vi "ColorSensor.vi"() -> ()   [LabVIEW 2016, in "ENED1100-UCBA-Sensor-Motor-Testing.lvrbt"]
uses:
  ENED1100-UCBA-Sensor-Motor-Testing.lvrbt
  <vilib>/NXT/Subs/LVHSConnector.ctl
  <vilib>/NXT/LegoClasses/BrickReference/BrickReference.lvclass
  <vilib>/NXT/Block Support/NXT_InputPort.ctl
  <vilib>/NXT/Subs/ColorSensorColors.ctl
  <vilib>/NXT/Dual Mode Library/Sensors/EV3_Color_Color.vi
panel:
  out "NXT/EV3 2":T1
  out "Detected Color":T2
  in  "Select Port Here":T3 items=["Port 1", "Port 2", "Port 3", "Port 4"]
  in  "NXT/EV3":T1
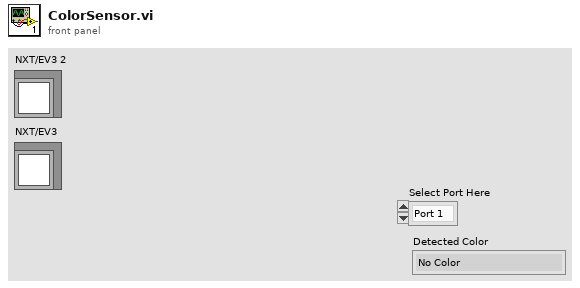
[diagram p1: front panel]
types:
  T1 = typedef "LVHSConnector.ctl" = refnum<class "BrickReference.lvclass">
  T2 = typedef "ColorSensorColors.ctl" = enum16{"No Color", "Black", "Blue", "Green", "Yellow", "Red", "White", "Brown"}
  T3 = typedef "NXT_InputPort.ctl" = u32
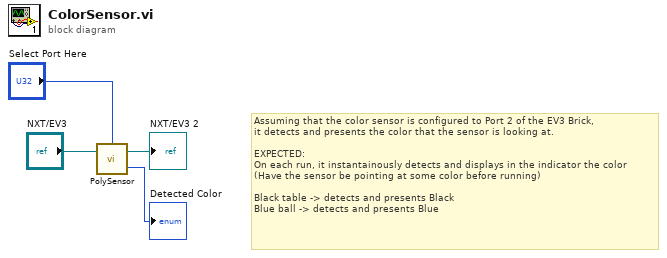
[diagram p0: block diagram]
diagram:
  # "Assuming that the color sensor is configured to Port 2 of the EV3 Brick,\nit detects and presents the color that the sensor is looking at.\n\nEXPECTED:\nOn each run, it instantainously detects and displays in the indicator the color\n(Have the sensor be pointing at some color before running)\n\nBlack table -> detects and presents Black\nBlue ball -> detects and presents Blue"
  n1 = call-poly <vilib>:"PolySensor.vi"("NXT/EV3"="NXT/EV3", "Port (Port 1)"="Select Port Here") -> ("Detected Color"=→"Detected Color":T2, "NXT/EV3"=→"NXT/EV3 2":T1)  [unwired: 1 in]
